vi "Log Data_PWM.vi"(0 "refnum in":refnum<file>, 1 "Temp (C)":dbl, 2 "Heater Status":bool, 3 "Set Point FB":i32 caption="Temp Set Point (C)", 4 "On/Off Set":bool, 5 "Error In":errorcluster, 9 "PWM":i32) -> (14 "refnum out":refnum<file>, 19 "Error Out":errorcluster)   [LabVIEW 2015]
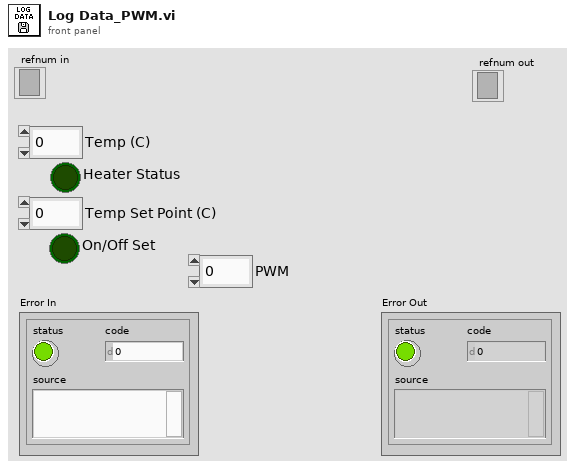
[diagram p1: front panel]
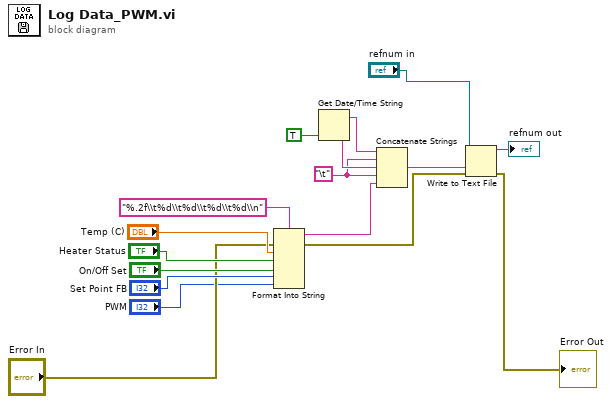
[diagram p0: block diagram]
diagram:
  w13 = "\t"
  n1 = Format Into String(format string="%.2f\\t%d\\t%d\\t%d\\t%d\\n", error in="Error In", "Temp (C)", "Heater Status", "On/Off Set", "Set Point FB", "PWM") -> (resulting string=w8:string, error out=w3:errorcluster)  [unwired: 1 in]
  n2 = Get Date/Time String(want seconds? (F)=TRUE) -> (date string=w16:string, time string=w15:string)  [unwired: 2 in]
  n3 = Concatenate Strings(w16, w13, w15, w13, w8) -> (w14:string)
  n4 = Write to Text File(file (use dialog)="refnum in", text=w14, error in=w3) -> (refnum out=→"refnum out":refnum<file>, error out=→"Error Out":errorcluster)  [unwired: 1 in, 1 out]
